vi "Take Control Panel Snapshot.vi"(8 "error in (no error)":errorcluster, 11 "Device in":refnum<class "Device.lvclass">) -> (0 "error out":errorcluster, 2 "Data":variant, 3 "Device out":refnum<class "Device.lvclass">)   [LabVIEW 2015, in "Device.lvclass"]
uses:
  Device.lvclass
  Write Controls Snapshot.vi
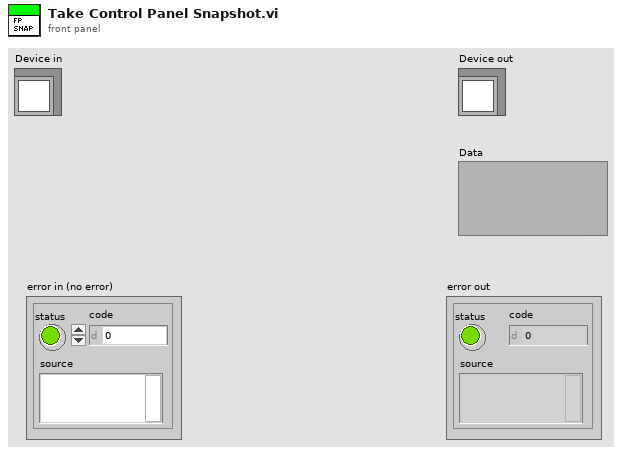
[diagram p1: front panel]
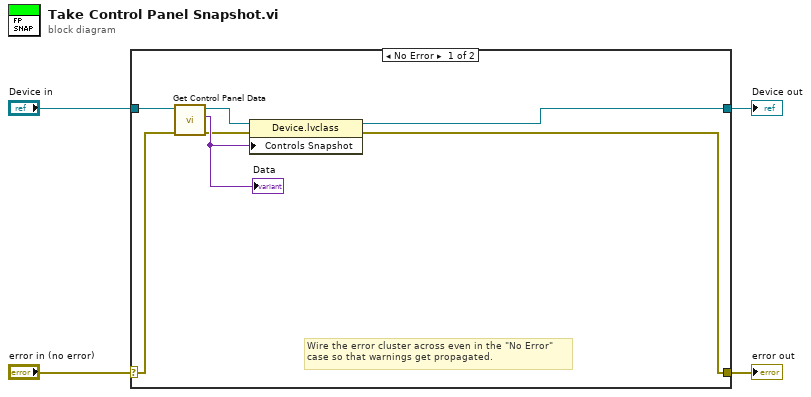
[diagram p0: block diagram]
diagram:
  n1 = case shown="No Error" "error in (no error)" {
    selector: "error in (no error)" -> [w9 w13]
    tunnel: [w5 w13] -> w3
    tunnel: [w8 w12] -> w1
    tunnel: "Device in" -> [w11 w12]
    frame No Error {
      # "Wire the error cluster across even in the \"No Error\"\ncase so that warnings get propagated."
      n2 = call-dynamic "Get Control Panel Data.vi"("error in (no error)"=w9, "Device in"=w11) -> ("error out"=w6:errorcluster, "Data"=w7:variant, "Device out"=w10:refnum<class "Device.lvclass">)  [unwired: 7 in]
      "Data" <- w7
      n3 = property class="Device.lvclass"(reference=w10, error in=w6, "Controls Snapshot"=w7) -> (reference out=w8:refnum<class "Device.lvclass">, error out=w5:errorcluster)
    }
    frame Error {
    }
  }
  "error out" <- w3
  "Device out" <- w1
